vi "colour generate VI.vi"() -> ()   [LabVIEW 2020]
panel:
  out "Colour":enum16{"green", "blue", "red", "yellow"}(ring)
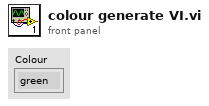
[diagram p1: front panel]
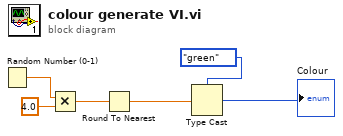
[diagram p0: block diagram]
diagram:
  n1 = Random Number (0-1)() -> (number: 0 to 1=w6:dbl)
  n2 = Multiply(x=w6, y=4.0) -> (x*y=w4:dbl)
  n3 = Round To Nearest(number=w4) -> (nearest integer value=w3:dbl)
  n4 = Type Cast(type=enum16{"green", "blue", "red", "yellow"}."green", x=w3) -> (*(type *) &x=→"Colour":enum16{"green", "blue", "red", "yellow"})
